vi "Do Command.vi"(6 "Actions In":refnum<class "Iteration Actions.lvclass">, 7 "Variables in":refnum<class "Variables.lvclass">, 8 "error in (no error)":errorcluster, 9 "Sequence Time":T1, 10 "VolatusAPI":refnum<class "VolatusAPI.lvclass">, 11 "Start Log Command in":refnum<class "Start Log Command.lvclass">) -> (0 "error out":errorcluster, 4 "Actions":refnum<class "Iteration Actions.lvclass">, 5 "Variables":refnum<class "Variables.lvclass">)   [LabVIEW 2020, in "VolatusSeq.lvlib" / "Start Log Command.lvclass"]
uses:
  Start Log Command.lvclass
  Variables/Variables.lvclass
  Volatus/VolatusAPI/VolatusAPI.lvclass
  Iteration Actions/Iteration Actions.lvclass
  lv-cdm/CDM-Config/ISO8601 Config.ctl
  lv-cdm/CDM-Config/Format.ctl
  lv-cdm/CDM-Config/Precision.ctl
  lv-cdm/CDM-Config/Timezone.ctl
  Start Log Command.lvclass/Start Log Command.ctl
  messages/StartLog/Class/Msg.lvclass/Msg.ctl
  Volatus/VolatusAPI/VolatusAPI.lvclass/VolatusAPI.ctl
  messages/StartLog/Class/Msg.lvclass
  C:/dev/lv20CE/relink/lv-protoc/LV-Proto/Message/Message.lvclass
  lv-cdm/CDM-Config/ISO-8601 Format Strings.vi
  lv-vecto/Vecto/TCPMessageService/Send Message.vi
  <vilib>/Utility/error.llb/Error Cluster From Error Code.vi
  lv-protoc/LV-Proto/Message/Message.lvclass
  lv-cdm/CDM-Config/CDM-Config.lvlib
  Sequence Time.ctl
  VolatusSeq.lvlib
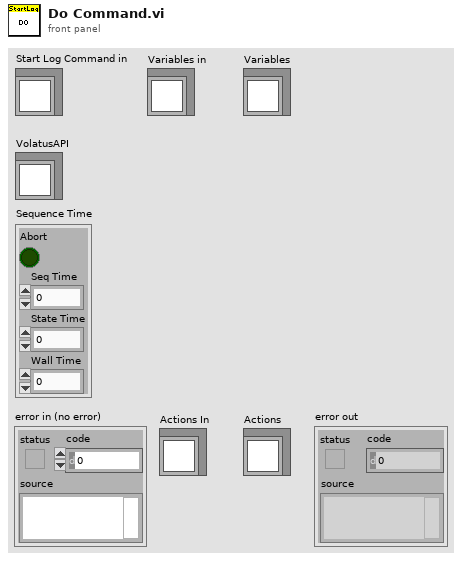
[diagram p1: front panel]
types:
  T1 = typedef "VolatusSeq.lvlib/Sequence Time.ctl" = cluster{"Abort":bool, "Seq Time":dbl, "State Time":dbl, "Wall Time":dbl}
  T2 = typedef "CDM-Config.lvlib/ISO8601 Config.ctl" = cluster{"Format":T3, "Precision":T4, "Timezone":T5}
  T3 = typedef "CDM-Config.lvlib/Format.ctl" = enum16{"Extended", "Basic"}
  T4 = typedef "CDM-Config.lvlib/Precision.ctl" = enum16{"Millisecond", "Second", "Minute", "Hour", "Day"}
  T5 = typedef "CDM-Config.lvlib/Timezone.ctl" = enum16{"UTC", "Local"}
  T6 = typedef "StartLog.lvlib/Data.ctl" = cluster{"series":string, "timestamp":string, "started_by":string, "groups":string[]}
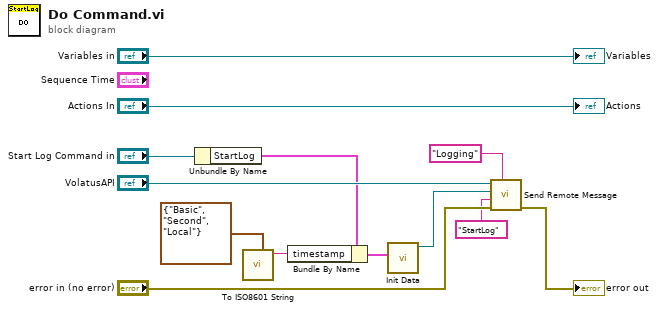
[diagram p0: block diagram]
diagram:
  n1 = Unbundle By Name("Start Log Command in") -> ("StartLog"=w7:T6)
  n2 = call "To ISO8601 String.vi"("Format Config"=T2 {"Format"=enum."Basic", "Precision"=enum."Second", "Timezone"=enum."Local"}) -> ("ISO 8601"=w5:string)  [unwired: 10 in]
  n3 = Bundle By Name(cluster=w7, "timestamp"=w5) -> (w4:T6)
  n4 = call "Init Data.vi"("Data"=w4) -> ("Msg out"=w3:refnum<class "Msg.lvclass">)  [unwired: 10 in]
  n5 = call "Send Remote Message.vi"("Target Name"="Logging", "error in (no error)"="error in (no error)", "Message Type"="StartLog", "Message"=w3, "VolatusAPI in"="VolatusAPI") -> ("error out"=→"error out":errorcluster)  [unwired: 5 in, 1 out]
  "Variables" <- "Variables in"
  "Actions" <- "Actions In"
